vi "Read Objects.vi"(8 "error in (no error)":errorcluster, 11 "device data model in":refnum<class "ICPCON ET Data Model.lvclass">) -> (0 "error out":errorcluster, 2 "objects":T1[](array[typedef]) {"Object ID" format="%x"}, 3 "device data model out":refnum<class "ICPCON ET Data Model.lvclass">)   [LabVIEW 2021, in "ICPCON ET Data Model.lvclass"]
doc: "Retrieves objects from the device model."
uses:
  ICPCON ET Data Model.lvclass
  Identification Parameters.ctl
  Device Data Model.lvclass
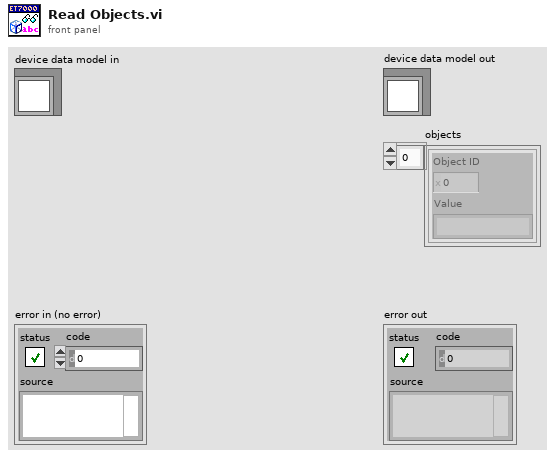
[diagram p1: front panel]
types:
  T1 = typedef "Device Data Model.lvclass/Identification Parameters.ctl" = cluster{"Object ID":u8, "Value":string}
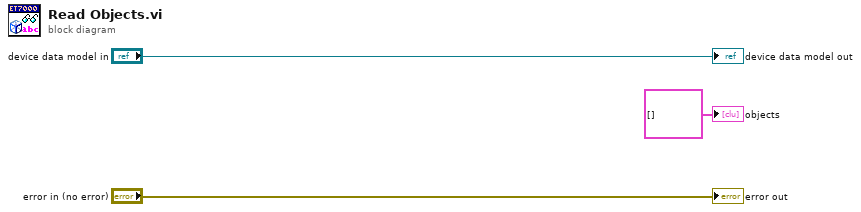
[diagram p0: block diagram]
diagram:
  "error out" <- "error in (no error)"
  "device data model out" <- "device data model in"
  "objects" <- T1[] [] ("objects")
